vi "Heise Barometric Pressure 901A Send Receive.vi"(8 "error in (no error)":errorcluster, 11 "VISA Refnum in":refnum<visa-resource-name>) -> (0 "error out":errorcluster, 1 "Barometric Data":string[](array[string]), 2 "Barometric Pressure (in Hg)":dbl, 3 "VISA Refnum out":refnum<visa-resource-name>, 5 "read buffer":string)   [LabVIEW 2023]
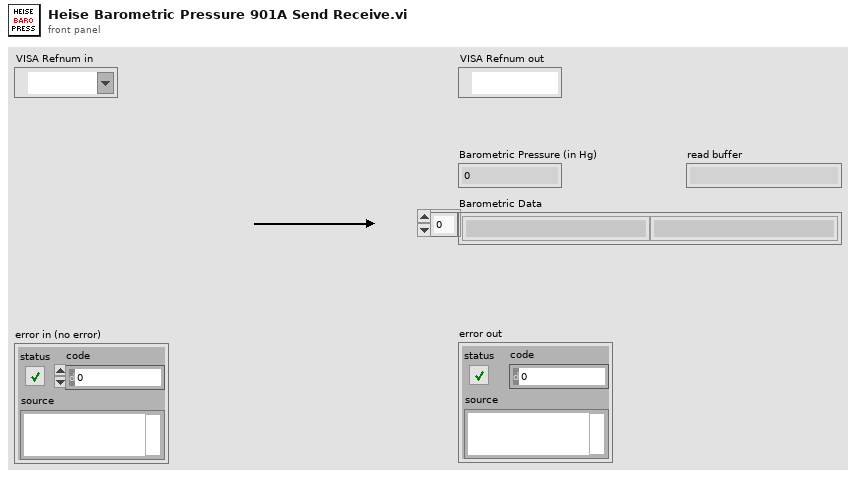
[diagram p1: front panel]
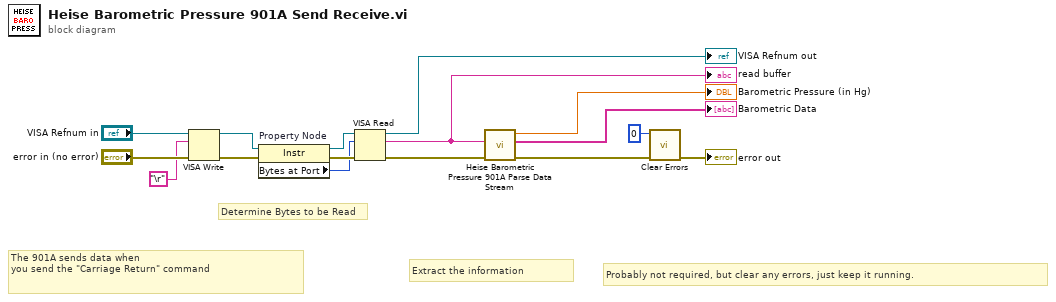
[diagram p0: block diagram]
diagram:
  # "Probably not required, but clear any errors, just keep it running."
  # "Extract the information"
  # "The 901A sends data when\nyou send the \"Carriage Return\" command"
  # "Determine Bytes to be Read"
  n1 = VISA Write(VISA resource name="VISA Refnum in", write buffer="\r", error in (no error)="error in (no error)") -> (VISA resource name out=w14:refnum<visa-resource-name>, error out=w12:errorcluster)  [unwired: 1 out]
  n2 = property on="Property Node" class="Instr"(reference=w14, error in=w12) -> (reference out=w13:refnum<visa-resource-name>, error out=w11:errorcluster, "Bytes at Port"=w10:u32)
  n3 = VISA Read(VISA resource name=w13, byte count=w10, error in (no error)=w11) -> (VISA resource name out=→"VISA Refnum out":refnum<visa-resource-name>, read buffer=w5:string, error out=w7:errorcluster)  [unwired: 1 out]
  "read buffer" <- w5
  n4 = call "Heise Barometric Pressure 901A Parse Data Stream.vi"("Error In"=w7, "Data Stream"=w5) -> ("Error Out"=w3:errorcluster, "Barometric Data"=→"Barometric Data":string[], "Barometric Pressure (in. Hg)"=→"Barometric Pressure (in Hg)":dbl)  [unwired: 7 in]
  n5 = call <vilib>:"Clear Errors.vi"("error in (no error)"=w3, "specific error code to clear (0: all)"=0) -> ("error out"=→"error out":errorcluster)  [unwired: 4 in, 1 out]
